vi "Metrolab_main.vi"() -> ()   [LabVIEW 2017]
panel:
  out "XY Graph":cluster{dbl[], dbl[]}(graph)
  in  "I_RF (A)":dbl=112.0
  in  "I_DC (A)":dbl=112.0
  out "Cycle #":i32
  in  "COMMENT":string="THM7025_zscan_practice"
  out "Graph (Bz)":cluster{timestamp[], dbl[]}(graph)={[timestamp(3708568369.45642 s since 1904-01-01), timestamp(3708568377.924761 s since 1904-01-01)], [0.25, 0.24]} caption="XY Graph"
  out "Graph (By)":cluster{timestamp[], dbl[]}(graph)={[timestamp(3708568369.45642 s since 1904-01-01), timestamp(3708568377.924761 s since 1904-01-01)], [-0.01, -0.01]} caption="XY Graph"
  in  "Stop":bool=TRUE
  out "Graph (Bx)":cluster{timestamp[], dbl[]}(graph)={[timestamp(3708568369.45642 s since 1904-01-01), timestamp(3708568377.924761 s since 1904-01-01)], [-0.02, -0.01]} caption="XY Graph"
  out "Z (mm) = 490 - L":dbl=378.0 format="%_5f"
  in  "L (mm)":dbl=112.0
  in  "Measure":bool
  out "File Error Out":errorcluster
  in  "base path":path=path "C:/LabVIEW/DATA/J-PARC_202107/B_measurement_0708"
  in  "error in (no error)":errorcluster caption="エラー入力（エラーなし）"
  out "error out":errorcluster caption="エラー出力" {"code" format="%.0x"}
  in  "VISA resource name":refnum<visa-resource-name>="COM4"
  out "Result (Bx, By, Bz,|B|)":dbl[](array[numeric])=[-0.24, -0.01, -0.01, 0.24]
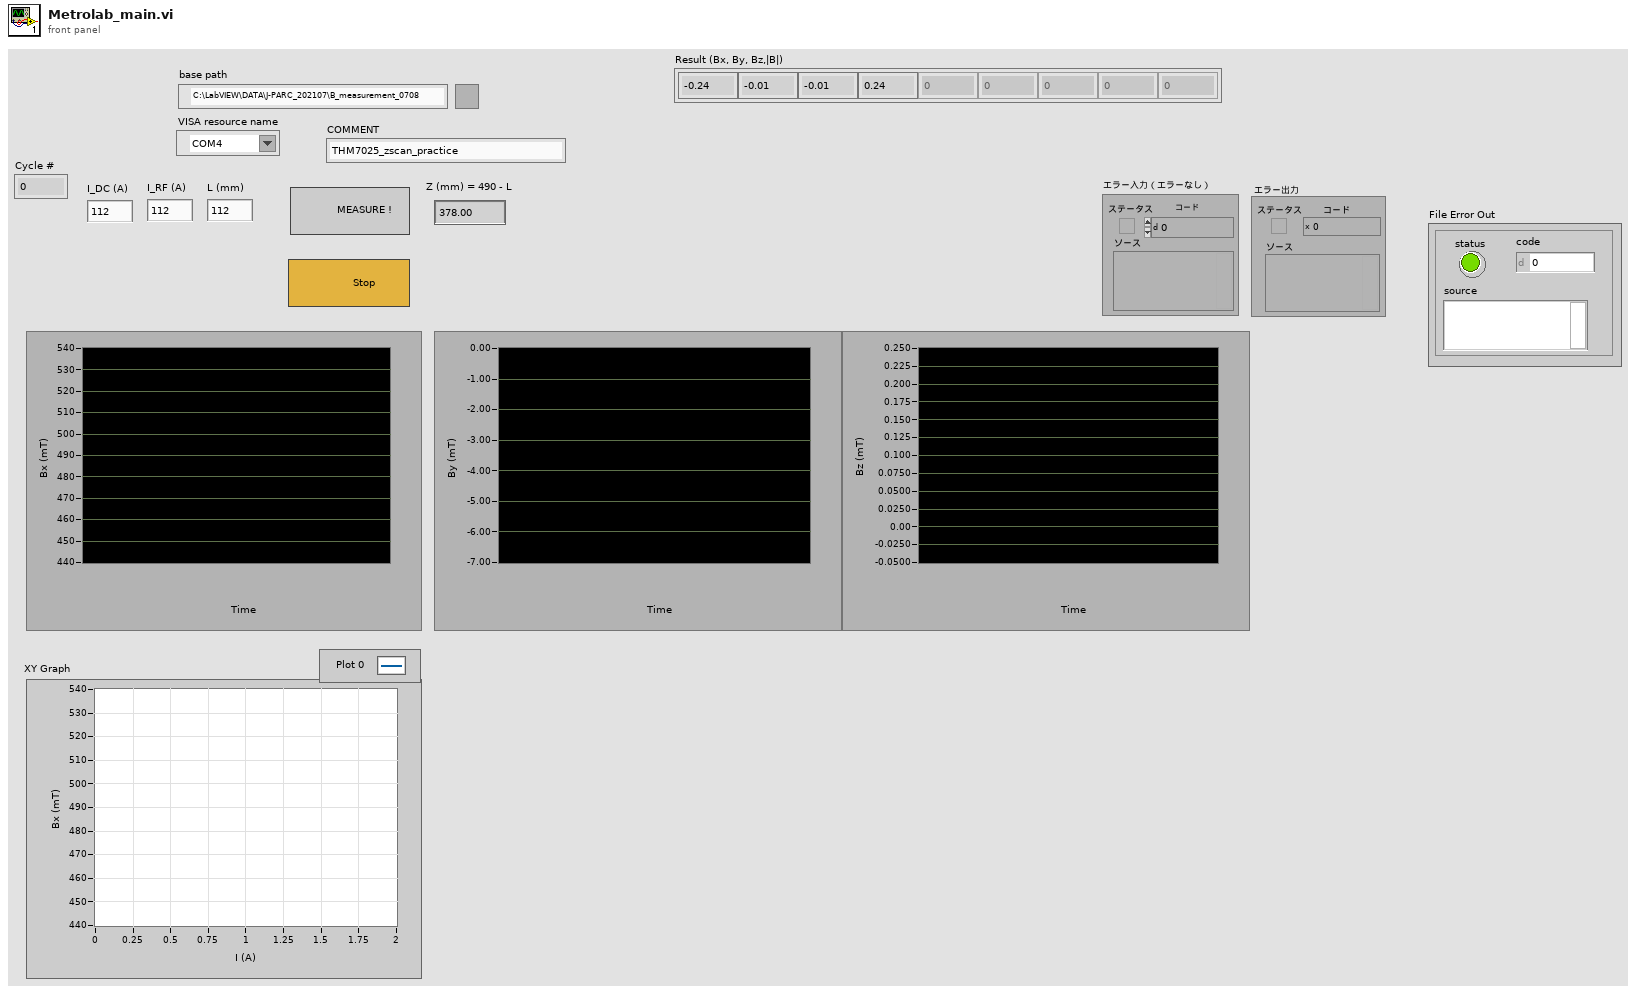
[diagram p1: front panel]
types:
  T1 = enum16{"open", "replace", "create", "open or create", "replace or create", "replace or create with confirmation"}
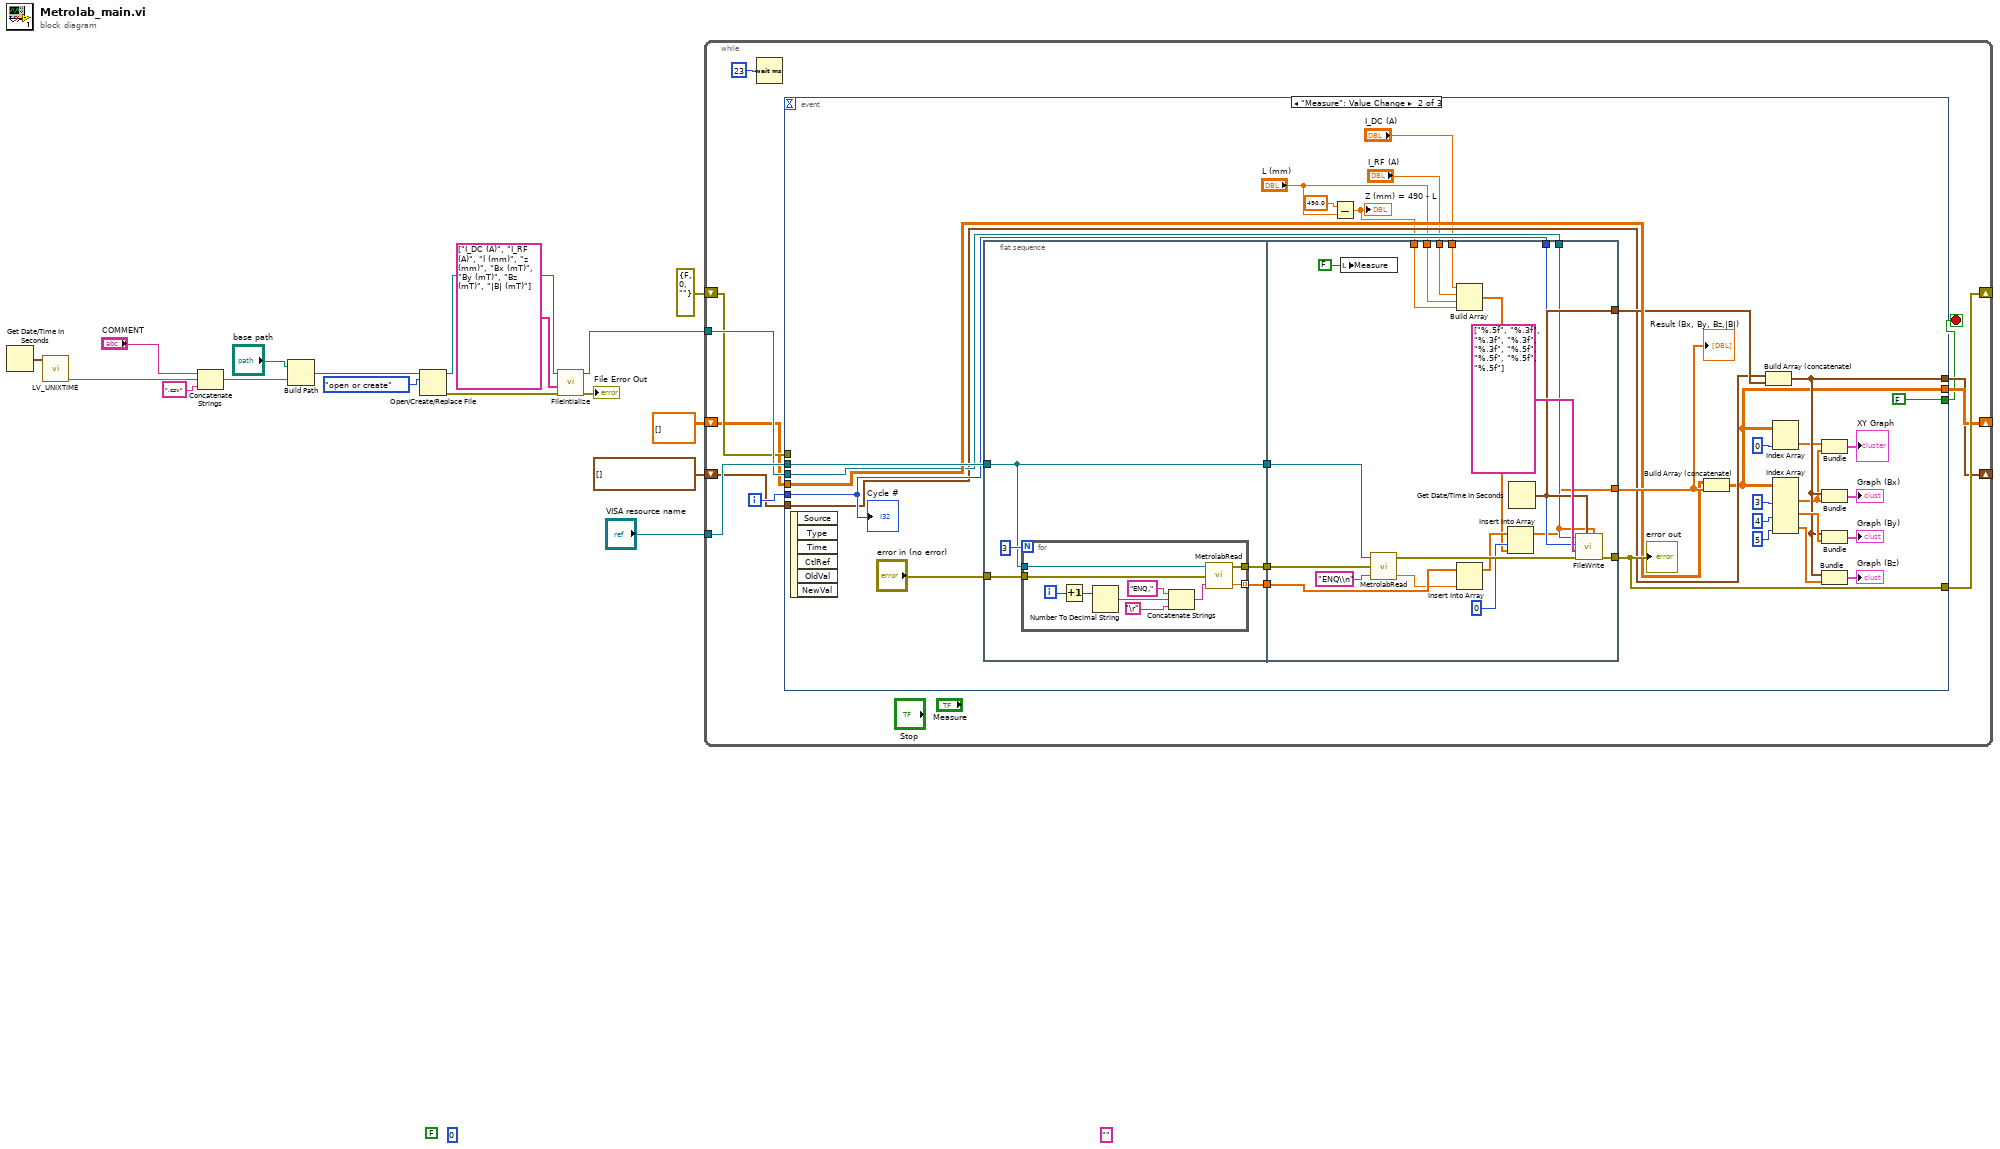
[diagram p0: block diagram]
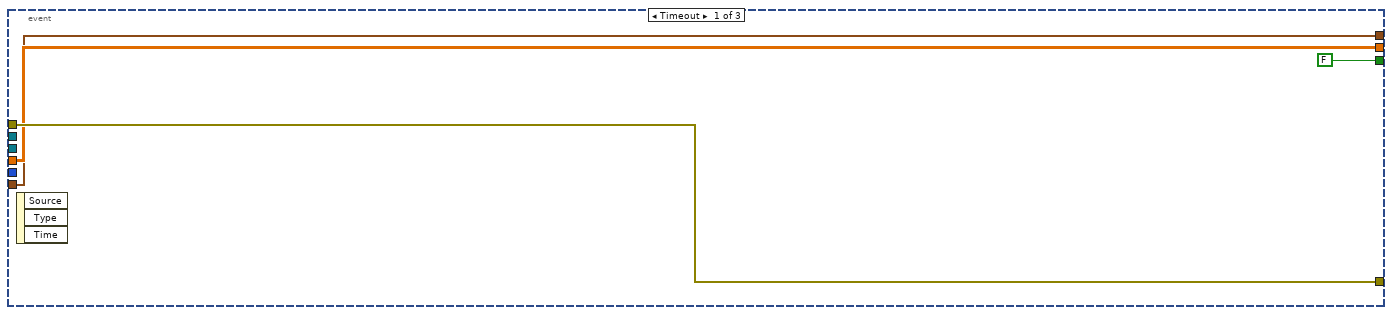
[diagram p2: hidden frame]
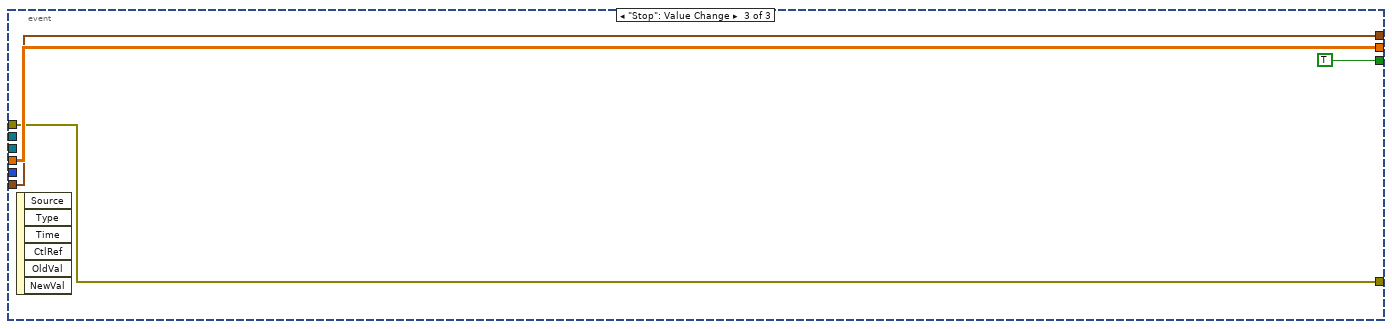
[diagram p3: hidden frame]
diagram:
  (unwired) FALSE ("status")
  (unwired) 0 ("code")
  (unwired) "" ("source")
  n1 = Get Date/Time In Seconds() -> (seconds since 1Jan1904=w14:timestamp)
  n2 = call "LV_UNIXTIME.vi"("current time"=w14) -> ("date/time string"=w11:string)  [unwired: 9 in, 1 out]
  n3 = Concatenate Strings("COMMENT", w11, ".csv" ("string")) -> (w9:string)
  n4 = Build Path(base path="base path", name or relative path=w9) -> (appended path=w13:path)
  n5 = Open/Create/Replace File(file path (use dialog)=w13, operation (0:open)=T1."open or create") -> (refnum out=w6:refnum<file>, error out=w7:errorcluster)  [unwired: 4 in, 1 out]
  n6 = call "FileIntialize.vi"("Error In"=w7, "Labels"=string[] ["I_DC (A)", "I_RF (A)", "l (mm)", "z (mm)", "Bx (mT)", "By (mT)", "Bz (mT)", "|B| (mT)"], "refnum in"=w6) -> ("Error Out"=→"File Error Out":errorcluster, "File Refnum"=w4:refnum<file>)  [unwired: 7 in]
  n7 = while {
    tunnel: "VISA resource name" -> [w27]
    tunnel: w4 -> [w26]
    shift-right: [w24] -> _
    shift-left: errorcluster {"status"=FALSE, "code"=0, "source"=""} ("Error Out") -> [w23]
    shift-right: [w21] -> _
    shift-left: dbl[][] [] -> [w22]
    shift-right: [w20] -> _
    shift-left: timestamp[] [] -> [w19]
    i -> [w25]
    stop <- w18 stop-if-true
    n8 = Wait (ms)(milliseconds to wait=u32 23) -> ()  [unwired: 1 out]
    n9 = event shown="[1] \"Measure\": Value Change" {
      selector: _ -> [_ _ _]
      dyn-events: _ -> [_ _ _]
      timeout: _ -> [_ _ _]
      tunnel: w27 -> [_ w60 _]
      tunnel: w26 -> [_ w51 _]
      tunnel: w25 -> [_ w50 _]
      tunnel: [w32 w58 w100] -> w24
      tunnel: w23 -> [w32 _ w100]
      tunnel: w22 -> [w31 w56 w102]
      tunnel: [w31 w37 w102] -> w21
      tunnel: [w29 w40 w101] -> w20
      tunnel: w19 -> [w29 w49 w101]
      tunnel: [FALSE ("Stop") FALSE ("Stop") TRUE ("Stop")] -> w18
      event Timeout {
        n10 = event-data() -> ()  [unwired: 1 in, 3 out]
      }
      event "Measure": Value Change {
        n11 = event-data() -> ()  [unwired: 1 in, 6 out]
        n12 = flat-sequence {
          tunnel: [w65] -> w64
          tunnel: [w68] -> w63
          tunnel: [w67] -> w62
          tunnel: "error in (no error)" -> [w66]
          tunnel: w60 -> [w65]
          tunnel: w64 -> [w99]
          tunnel: w63 -> [w98]
          tunnel: w62 -> [w96]
          tunnel: [w80] -> w57
          tunnel: [w92] -> w58
          tunnel: [w91] -> w52
          tunnel: w51 -> [w90]
          tunnel: w50 -> [w89]
          tunnel: "L (mm)" -> [w88]
          tunnel: w46 -> [w87]
          tunnel: "I_DC (A)" -> [w83]
          tunnel: "I_RF (A)" -> [w82]
          frame #0 {
            n13 = for {
              N: 3 -> [_]
              tunnel: w65 -> [w79]
              tunnel: [w75] -> w67 mode=indexing
              tunnel: [w71] -> w68
              tunnel: w66 -> [w70]
              i -> [w72]
              n14 = Increment(x=w72) -> (x+1=w73:i32)
              n15 = Number To Decimal String(number=w73) -> (decimal integer string=w76:string)  [unwired: 1 in]
              n16 = Concatenate Strings("ENQ,", w76, "\r") -> (w77:string)
              n17 = call "MetrolabRead.vi"("Input string"=w77, "error in (no error)"=w70, "VISA resource name"=w79) -> ("B value [mT]"=w75:dbl, "error out"=w71:errorcluster)  [unwired: 1 out]
            }
          }
          frame #1 {
            n18 = local write "Measure"(FALSE ("Value (Signaling)")) -> ()
            n19 = call "MetrolabRead.vi"("Input string"="ENQ\\n", "error in (no error)"=w98, "VISA resource name"=w99) -> ("B value [mT]"=w95:dbl, "error out"=w93:errorcluster)  [unwired: 1 out]
            n20 = Build Array(w83, w82, w88, w87) -> (w81:dbl[])
            n21 = Insert Into Array(array=w96, new element=w95) -> (w84:dbl[])  [unwired: 1 in]
            n22 = Insert Into Array(array=w84, index=0, new element=w81) -> (w80:dbl[])
            n23 = Get Date/Time In Seconds() -> (seconds since 1Jan1904=w91:timestamp)
            n24 = call "FileWrite.vi"("DataArray"=w80, "Time Stamp"=w91, "Error In"=w93, "FileFormat"=string[] ["%.5f", "%.3f", "%.3f", "%.3f", "%.3f", "%.5f", "%.5f", "%.5f", "%.5f"], "Index"=w89, "refnum in"=w90) -> ("Error Out"=w92:errorcluster)  [unwired: 4 in, 1 out]
          }
        }
        n25 = Subtract(x=490.0, y="L (mm)") -> (x-y=w46:dbl)
        "Z (mm) = 490 - L" <- w46
        n26 = Build Array (concatenate)(w56, w57) -> (w37:dbl[][])
        n27 = Build Array (concatenate)(w49, w52) -> (w40:timestamp[])
        n28 = Index Array(array=w37, index (col)=0 ("disabled index (col)")) -> (element=w35:dbl[])  [unwired: 1 in]
        n29 = Index Array(array=w37, index (col) #1=3 ("disabled index (col)"), index (col) #2=4 ("disabled index (col)"), index (col) #3=5 ("disabled index (col)")) -> (element #1=w34:dbl[], element #2=w42:dbl[], element #3=w41:dbl[])  [unwired: 3 in]
        n30 = Bundle(w35, w34) -> (→"XY Graph":cluster{dbl[], dbl[]})  [unwired: 1 in]
        n31 = Bundle(w40, w34) -> (→"Graph (Bx)":cluster{timestamp[], dbl[]})  [unwired: 1 in]
        n32 = Bundle(w40, w42) -> (→"Graph (By)":cluster{timestamp[], dbl[]})  [unwired: 1 in]
        n33 = Bundle(w40, w41) -> (→"Graph (Bz)":cluster{timestamp[], dbl[]})  [unwired: 1 in]
        "Result (Bx, By, Bz,|B|)" <- w57
        "error out" <- w58
        "Cycle #" <- w50
      }
      event "Stop": Value Change {
        n34 = event-data() -> ()  [unwired: 1 in, 6 out]
      }
    }
  }
